vi "Initialize Transceiver.vi"(7 "transceiver settings":T1, 8 "error in (no error)":errorcluster, 9 "Transfer Groups Configurations":T2[](array[typedef]) {"Transfers"."channel configurations"."buffer offset" format="%d bytes"}, 10 "component classes":refnum<class>[](array[class]), 11 "Plugin in":refnum<class "Plugin.lvclass">) -> (0 "error out":errorcluster, 2 "Transceiver":refnum<class "Transceiver.lvclass">, 3 "Plugin out":refnum<class "Plugin.lvclass">)   [LabVIEW 2017, in "DSF Core.lvlib" / "Plugin.lvclass"]
uses:
  Plugin.lvclass
  DSF Configuration API/Public/Controls/DSF Engine Transfer Group Configuration.ctl
  DSF Configuration API/Public/Controls/DSF Direction.ctl
  DSF Configuration API/Public/Controls/DSF Timing Info.ctl
  DSF Configuration API/Public/Controls/DSF Engine Transfer Configuration.ctl
  DSF Configuration API/Public/Controls/DSF Byte Order.ctl
  DSF Configuration API/Public/Controls/DSF Engine Channel Configuration.ctl
  DSF Configuration API/Public/Controls/DSF Data Type.ctl
  DSF Configuration API/Public/Controls/DSF Settings Info.ctl
  Transceiver/Transceiver.lvclass
  DSF Core.lvlib
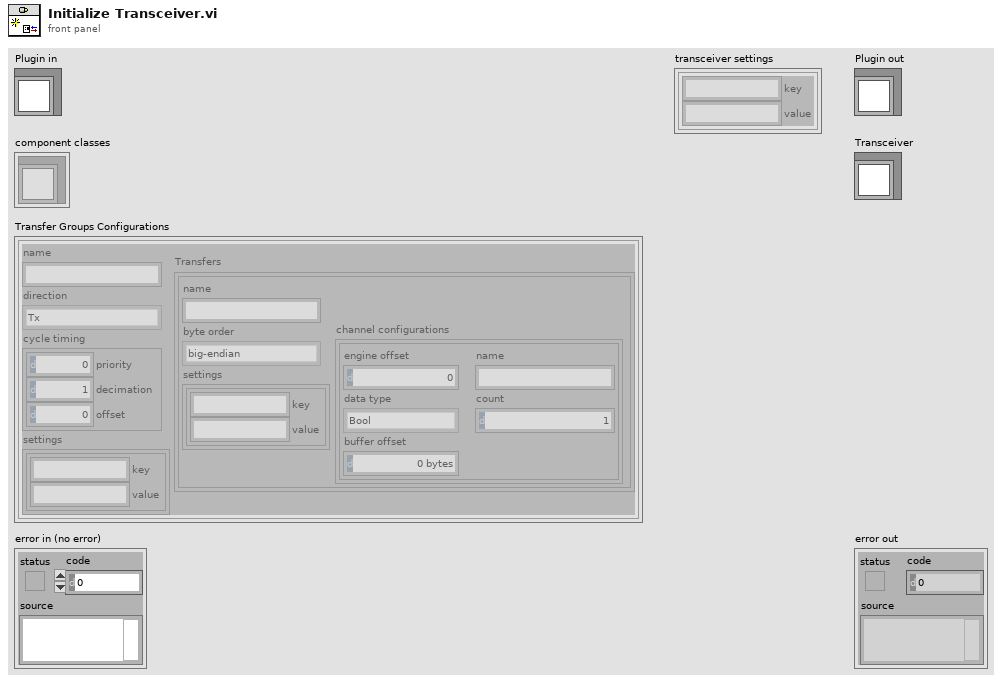
[diagram p1: front panel]
types:
  T1 = typedef "DSF Core.lvlib/DSF Settings Info.ctl" = cluster{"key":string, "value":string}[]
  T2 = typedef "DSF Core.lvlib/DSF Engine Transfer Group Configuration.ctl" = cluster{"name":string, "direction":T3, "cycle timing":T4, "Transfers":T5[], "settings":T1}
  T3 = typedef "DSF Core.lvlib/DSF Direction.ctl" = enum8{"Tx", "Rx"}
  T4 = typedef "DSF Core.lvlib/DSF Timing Info.ctl" = cluster{"priority":u64, "decimation":u64, "offset":u64}
  T5 = typedef "DSF Core.lvlib/DSF Engine Transfer Configuration.ctl" = cluster{"name":string, "byte order":T6, "channel configurations":T7[], "settings":T1}
  T6 = typedef "DSF Core.lvlib/DSF Byte Order.ctl" = enum8{"big-endian", "little-endian"}
  T7 = typedef "DSF Core.lvlib/DSF Engine Channel Configuration.ctl" = cluster{"engine offset":u64, "name":string, "data type":T8, "count":u64, "buffer offset":u64}
  T8 = typedef "DSF Core.lvlib/DSF Data Type.ctl" = enum8{"Bool", "SGL", "DBL", "I8", "I16", "I32", "I64", "U8", "U16", "U32", "U64"}
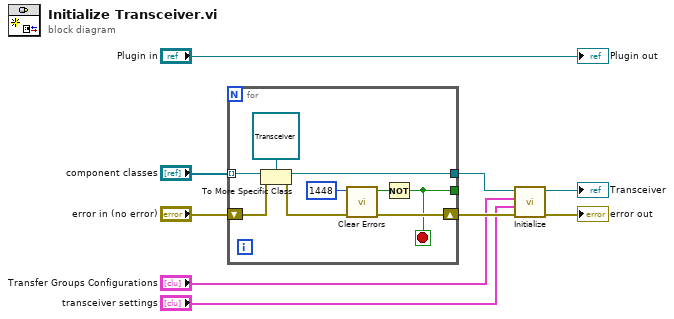
[diagram p0: block diagram]
diagram:
  n1 = for {
    tunnel: "component classes" -> [w17] mode=indexing
    tunnel: [w16] -> w5
    shift-right: [w13] -> w6
    shift-left: "error in (no error)" -> [w12]
    tunnel: [w10] -> _
    stop <- w10 stop-if-true
    n2 = To More Specific Class(target class=refnum<class "Transceiver.lvclass"> refnum ("DSF.Engine.lvlib:Transceiver"), reference=w17, error in=w12) -> (specific class reference=w16:refnum<class "Transceiver.lvclass">, error out=w14:errorcluster)
    n3 = call <vilib>:"Clear Errors.vi"("error in (no error)"=w14, "specific error code to clear (0: all)"=1448) -> ("error out"=w13:errorcluster, "specific error cleared?"=w11:bool)  [unwired: 4 in]
    n4 = Not(x=w11) -> (.not. x?=w10:bool)
  }
  n5 = call-dynamic "Initialize.vi"("error in (no error)"=w6, "transceiver settings"="transceiver settings", "Transfer Groups Configurations"="Transfer Groups Configurations", "Transceiver in"=w5) -> ("error out"=→"error out":errorcluster, "Transceiver out"=→"Transceiver":refnum<class "Transceiver.lvclass">)  [unwired: 6 in]
  "Plugin out" <- "Plugin in"
